vi "Set Force Table Settings.vi"(10 "Force Table Settings":T1 {"Entries"."Force Set Points"."Axial Force" format="%.4f"; "Entries"."Force Set Points"."Lateral Force" format="%.4f"}, 11 "Model in":refnum<class "Model.lvclass">) -> (3 "Model out":refnum<class "Model.lvclass">)   [LabVIEW 2016]
uses:
  Model.lvclass
  Typedefs/ForcePair.ctl
  Typedefs/ForceTableEntry.ctl
  Typedefs/ForceTableSettings.ctl
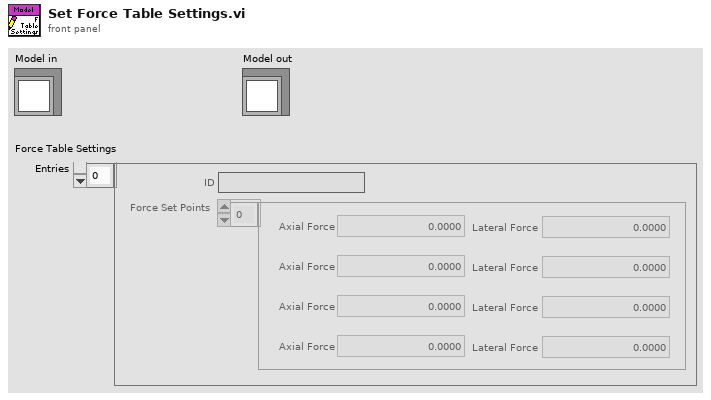
[diagram p1: front panel]
types:
  T1 = typedef "ForceTableSettings.ctl" = cluster{"Entries":T2[]}
  T2 = typedef "ForceTableEntry.ctl" = cluster{"ID":string, "Force Set Points":T3[]}
  T3 = typedef "ForcePair.ctl" = cluster{"Axial Force":dbl, "Lateral Force":dbl}
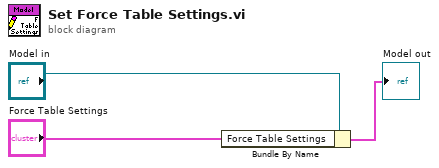
[diagram p0: block diagram]
diagram:
  n1 = Bundle By Name(cluster="Model in", "Force Table Settings"="Force Table Settings") -> (→"Model out":cluster{})
